vi "1.1 индикар полки.vi"(11 "appended array":bool[](array[boolean])) -> (3 "текущее положение":string)   [LabVIEW 2016, in "Library.lvlib"]
uses:
  Granule-2000AT/PC/Library.lvlib
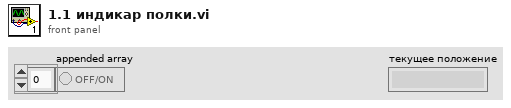
[diagram p1: front panel]
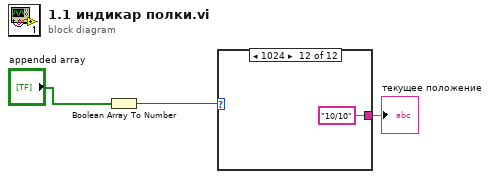
[diagram p0: block diagram]
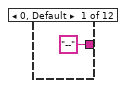
[diagram p2: hidden frame]
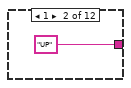
[diagram p3: hidden frame]
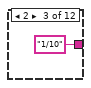
[diagram p4: hidden frame]
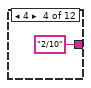
[diagram p5: hidden frame]
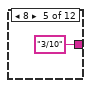
[diagram p6: hidden frame]
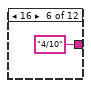
[diagram p7: hidden frame]
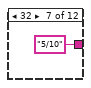
[diagram p8: hidden frame]
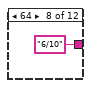
[diagram p9: hidden frame]
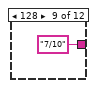
[diagram p10: hidden frame]
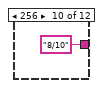
[diagram p11: hidden frame]
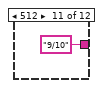
[diagram p12: hidden frame]
diagram:
  n1 = Boolean Array To Number(Boolean array="appended array") -> (number=w2:u32)
  n2 = case shown="1024" w2 {
    tunnel: ["--" "UP" "1/10" "2/10" "3/10" "4/10" "5/10" "6/10" "7/10" "8/10" "9/10" "10/10"] -> w1
    frame 0, Default {
    }
    frame 1 {
    }
    frame 2 {
    }
    frame 4 {
    }
    frame 8 {
    }
    frame 16 {
    }
    frame 32 {
    }
    frame 64 {
    }
    frame 128 {
    }
    frame 256 {
    }
    frame 512 {
    }
    frame 1024 {
    }
  }
  "текущее положение" <- w1
